vi "waveform format test.vi"() -> ()   [LabVIEW 2024]
panel:
  in  "Numeric 2":i32
  out "Array 2":i32[](array[numeric])
  in  "Numeric":i32
  in  "Array":waveform(dbl)[](array[waveform])
  out "Stream Response Graph":waveform(dbl)[](graph)
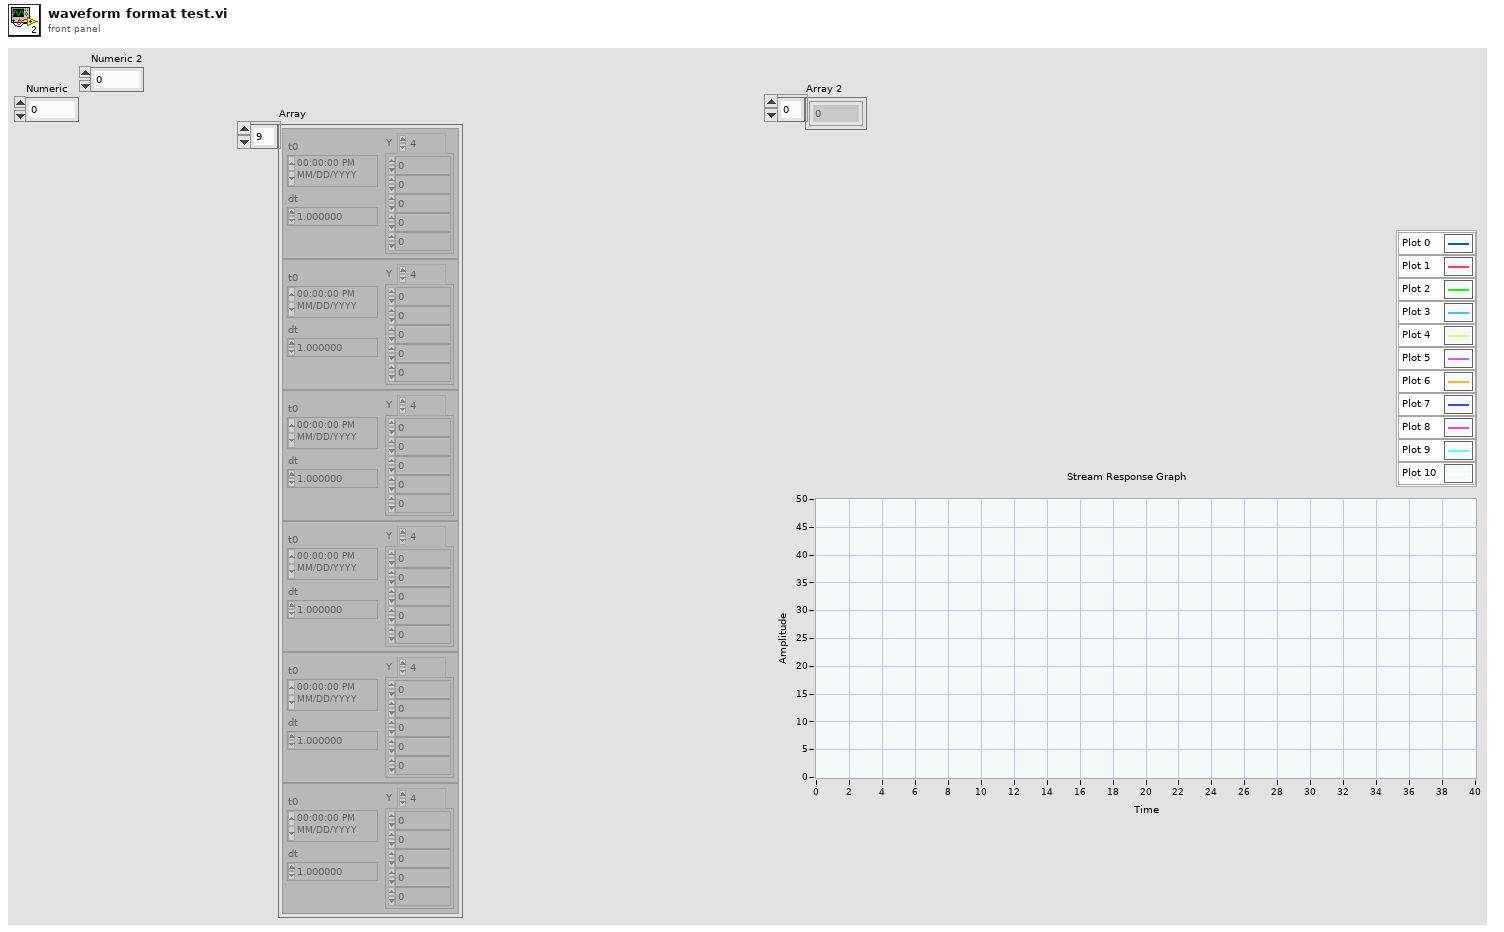
[diagram p1: front panel]
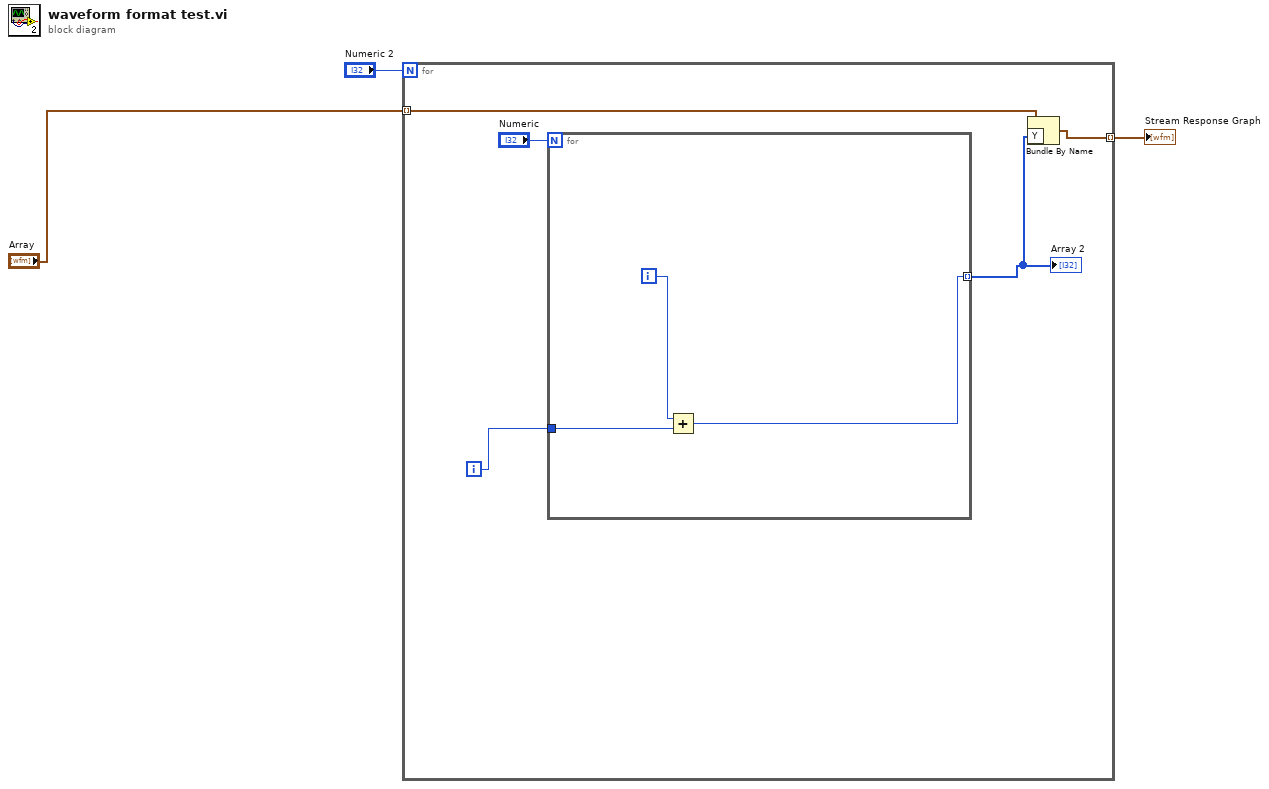
[diagram p0: block diagram]
diagram:
  n1 = for {
    N: "Numeric 2" -> [_]
    tunnel: "Array" -> [w7] mode=indexing
    tunnel: [w4] -> w2 mode=indexing
    i -> [w5]
    n2 = for {
      N: "Numeric" -> [_]
      tunnel: [w9] -> w6 mode=indexing
      tunnel: w5 -> [w11]
      i -> [w10]
      n3 = Add(x=w10, y=w11) -> (x+y=w9:i32)
    }
    "Array 2" <- w6
    n4 = Bundle By Name(cluster=w7, "Y"=w6) -> (w4:waveform(dbl))
  }
  "Stream Response Graph" <- w2
